vi "Read Excel (xlsx).vi"(7 "Excel._SheetName":string="Sheet1", 8 "error in (no error)":errorcluster, 11 "File Path Control":path) -> (0 "error out":errorcluster, 3 "data":string[][](array[string]))   [LabVIEW 2020]
panel:
  out "Array":string[](array[string])
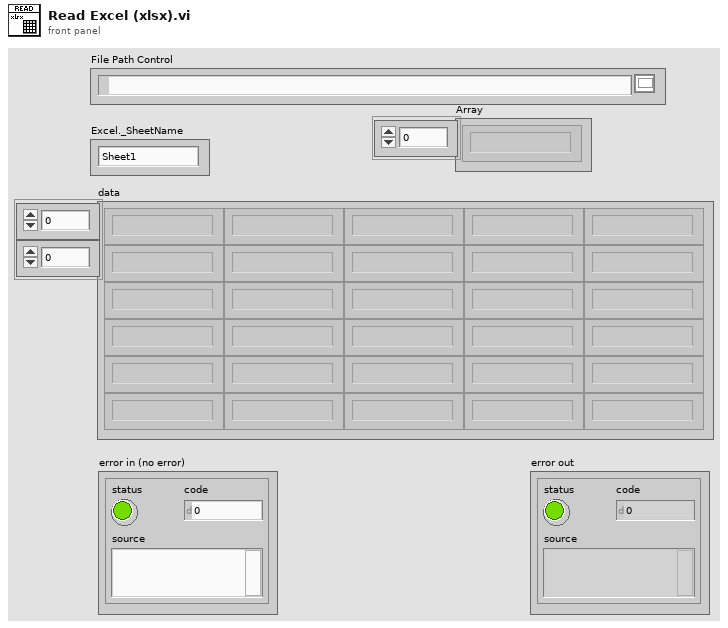
[diagram p1: front panel]
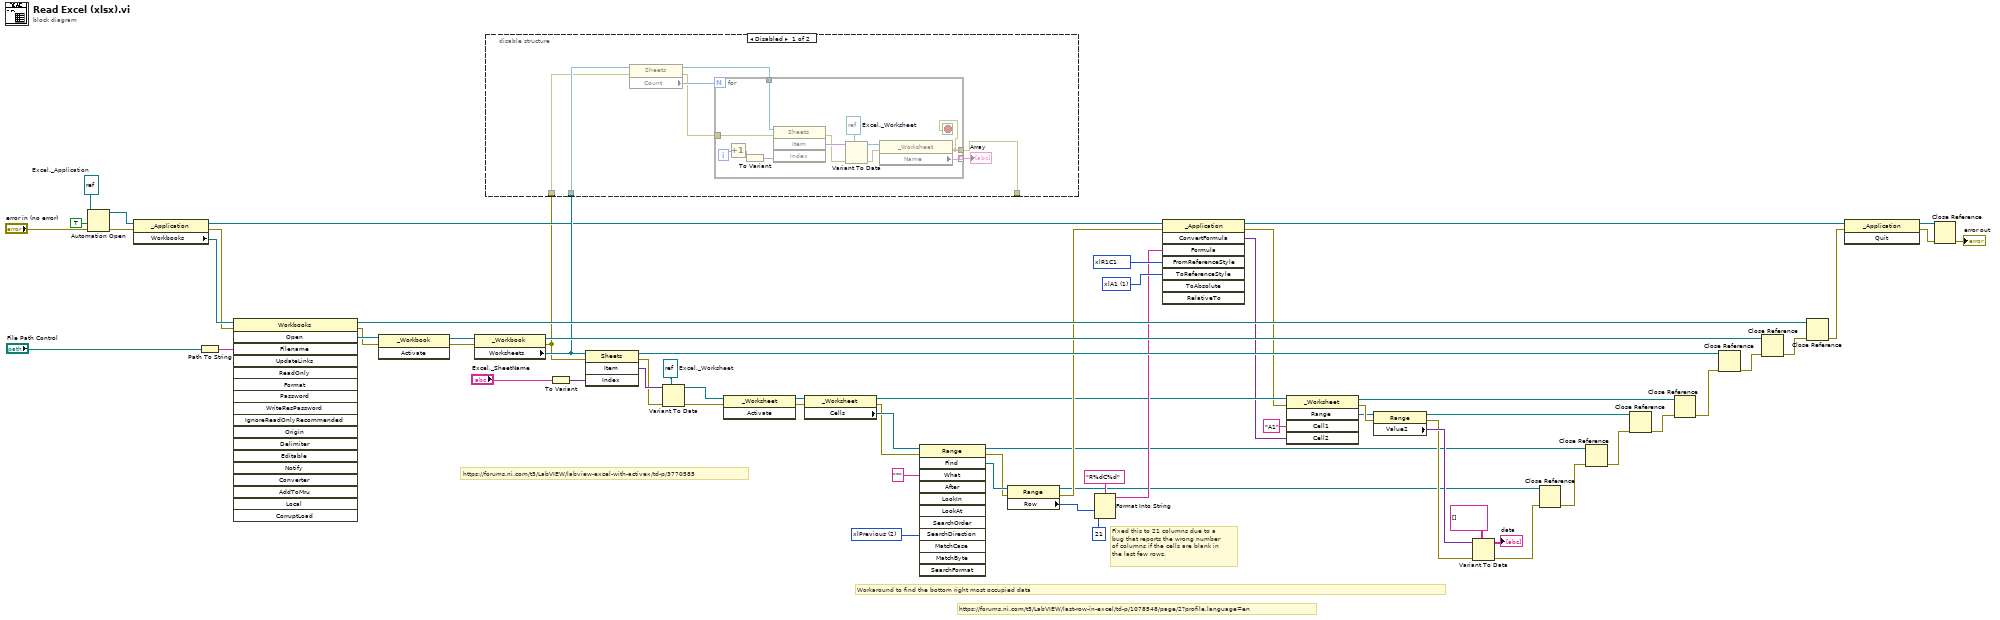
[diagram p0: block diagram]
diagram:
  w24 = 1 items=["xlA1"=1, "xlR1C1"=-4150] ("FromReferenceStyle")
  w25 = -4150 items=["xlA1"=1, "xlR1C1"=-4150] ("FromReferenceStyle")
  w29 = 2 items=["xlNext"=1, "xlPrevious"=2] ("SearchDirection")
  w56 = refnum<k7> refnum  # Excel._Worksheet
  w66 = refnum<k7> refnum  # Excel._Application
  # "Fixed this to 21 columns due to a bug that reports the wrong number of columns if the cells are blank in the last few rows."
  # "https://forums.ni.com/t5/LabVIEW/last-row-in-excel/td-p/1078548/page/2?profile.language=en"
  # "Workaround to find the bottom right most occupied data"
  # "https://forums.ni.com/t5/LabVIEW/labview-excel-with-activex/td-p/3770585"
  n1 = Automation Open(error in (no error)="error in (no error)", Automation Refnum=w66, 9:TRUE ("open new instance (false)")) -> (Automation Refnum=w42:refnum<k7>, error out=w65:errorcluster)  [unwired: 1 in]
  n2 = property class="_Application"(reference=w42, error in=w65) -> (reference out=w20:refnum<k7>, error out=w40:errorcluster, "Workbooks"=w64:refnum<k7>)
  n3 = Path To String(path="File Path Control") -> (string=w63:string)
  n4 = invoke class="Workbooks" method="Open"(reference=w64, error in=w40, "Filename"=w63) -> (reference out=w45:refnum<k7>, error out=w55:errorcluster, "Open"=w61:refnum<k7>)  [unwired: 15 in, 15 out]
  n5 = invoke class="_Workbook" method="Activate"(reference=w61, error in=w55) -> (reference out=w60:refnum<k7>, error out=w54:errorcluster)  [unwired: 1 in, 1 out]
  n6 = property class="_Workbook"(reference=w60, error in=w54) -> (reference out=w35:refnum<k7>, error out=w17:errorcluster, "Worksheets"=w33:refnum<k7>)
  n7 = disable-structure shown="Disabled" {
    disable-tunnel: w33 -> [w74 _]
    disable-tunnel: w17 -> [w70 w87]
    disable-tunnel: [w68 w87] -> _
    frame Disabled {
      n8 = property class="Sheets"(reference=w74, error in=w70) -> (reference out=w72:refnum<k7>, error out=w69:errorcluster, "Count"=w73:i32)
      n9 = for {
        N: w73 -> [_]
        tunnel: w72 -> [w86]
        tunnel: [w81] -> w71 mode=indexing
        tunnel: w69 -> [w80]
        tunnel: [w77] -> w68
        i -> [w76]
        stop <- w77 stop-if-true
        w84 = refnum<k7> refnum  # Excel._Worksheet
        n10 = Increment(x=w76) -> (x+1=w75:i32)
        n11 = To Variant(anything=w75) -> (Variant=w85:variant)
        n12 = invoke class="Sheets" method="Item"(reference=w86, error in=w80, "Index"=w85) -> (error out=w79:errorcluster, "Item"=w83:variant)  [unwired: 1 in, 2 out]
        n13 = Variant To Data(error in=w79, type=w84, Variant=w83) -> (data=w82:refnum<k7>, error out=w78:errorcluster)
        n14 = property class="_Worksheet"(reference=w82, error in=w78) -> (error out=w77:errorcluster, "Name"=w81:string)  [unwired: 1 out]
      }
      "Array" <- w71
    }
    frame Enabled {
    }
  }
  n15 = To Variant(anything="Excel._SheetName") -> (Variant=w59:variant)
  n16 = invoke class="Sheets" method="Item"(reference=w33, error in=w17, "Index"=w59) -> (reference out=w34:refnum<k7>, error out=w53:errorcluster, "Item"=w57:variant)  [unwired: 1 in, 1 out]
  n17 = Variant To Data(error in=w53, type=w56, Variant=w57) -> (data=w52:refnum<k7>, error out=w51:errorcluster)
  n18 = invoke class="_Worksheet" method="Activate"(reference=w52, error in=w51) -> (reference out=w44:refnum<k7>, error out=w43:errorcluster)  [unwired: 1 in, 1 out]
  n19 = property class="_Worksheet"(reference=w44, error in=w43) -> (reference out=w15:refnum<k7>, error out=w31:errorcluster, "Cells"=w32:refnum<k7>)
  n20 = invoke class="Range" method="Find"(reference=w32, error in=w31, "What"="*", "SearchDirection"=w29) -> (reference out=w8:refnum<k7>, error out=w21:errorcluster, "Find"=w28:refnum<k7>)  [unwired: 8 in, 9 out]
  n21 = property class="Range"(reference=w28, error in=w21) -> (reference out=w4:refnum<k7>, error out=w16:errorcluster, "Row"=w26:i32)
  n22 = Format Into String(format string="R%dC%d", w26, 21 ("input 2")) -> (resulting string=w18:string)  [unwired: 2 in, 1 out]
  n23 = invoke class="_Application" method="ConvertFormula"(reference=w20, error in=w16, "Formula"=w18, "FromReferenceStyle"=w25, "ToReferenceStyle"=w24) -> (reference out=w19:refnum<k7>, error out=w12:errorcluster, "ConvertFormula"=w13:variant)  [unwired: 3 in, 5 out]
  n24 = invoke class="_Worksheet" method="Range"(reference=w15, error in=w12, "Cell1"="A1" ("format string"), "Cell2"=w13) -> (reference out=w14:refnum<k7>, error out=w11:errorcluster, "Range"=w10:refnum<k7>)  [unwired: 1 in, 2 out]
  n25 = property class="Range"(reference=w10, error in=w11) -> (reference out=w5:refnum<k7>, error out=w9:errorcluster, "Value2"=w22:variant)
  n26 = Variant To Data(error in=w9, type=string[][] [], Variant=w22) -> (data=→"data":string[][], error out=w3:errorcluster)
  n27 = Close Reference(reference=w4, error in (no error)=w3) -> (error out=w2:errorcluster)
  n28 = Close Reference(reference=w8, error in (no error)=w2) -> (error out=w7:errorcluster)
  n29 = Close Reference(reference=w5, error in (no error)=w7) -> (error out=w6:errorcluster)
  n30 = Close Reference(reference=w14, error in (no error)=w6) -> (error out=w48:errorcluster)
  n31 = Close Reference(reference=w34, error in (no error)=w48) -> (error out=w47:errorcluster)
  n32 = Close Reference(reference=w35, error in (no error)=w47) -> (error out=w46:errorcluster)
  n33 = Close Reference(reference=w45, error in (no error)=w46) -> (error out=w38:errorcluster)
  n34 = invoke class="_Application" method="Quit"(reference=w19, error in=w38) -> (reference out=w39:refnum<k7>, error out=w37:errorcluster)  [unwired: 1 in, 1 out]
  n35 = Close Reference(reference=w39, error in (no error)=w37) -> (error out=→"error out":errorcluster)
